vi "QTrkGenerateSampleFromLUT.vi"(0 "Width":i32=80, 1 "Height":i32=80, 2 "position":cluster{"x":sgl, "y":sgl}={"x"=40.0, "y"=40.0}, 3 "LUT":sgl[][](array[numeric]), 4 "magnification":sgl=1.0, 5 "LUT radii":cluster{"min":sgl, "max":sgl}={"min"=0.0, "max"=40.0}, 7 "z":sgl=10.0, 9 "photoncountpp":sgl) -> (14 "image":sgl[][](array[numeric]))   [LabVIEW 2011]
uses:
  QTrkDLL.vi
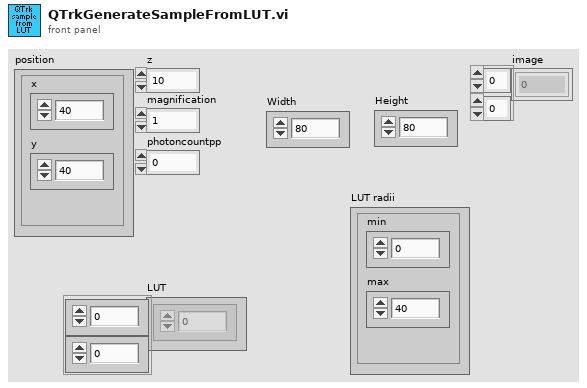
[diagram p1: front panel]
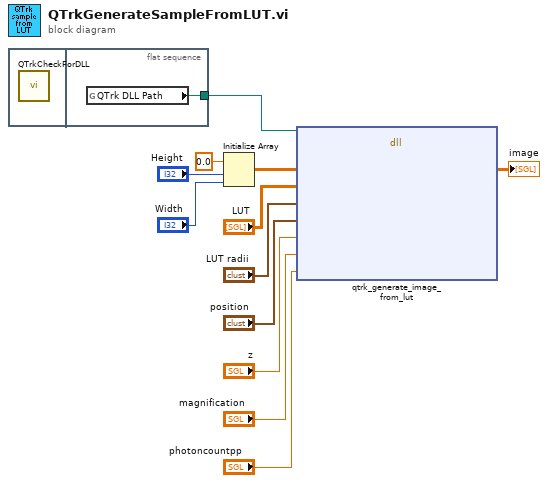
[diagram p0: block diagram]
diagram:
  n1 = flat-sequence {
    tunnel: [w13] -> w1
    frame #0 {
      n2 = call "QTrkCheckForDLL.vi"() -> ()  [unwired: 12 in]
    }
    frame #1 {
      n3 = global read "QTrkDLL.vi" "QTrk DLL Path"() -> (w13:path)
    }
  }
  n4 = Initialize Array(sgl 0.0 ("element"), "Height", "Width") -> (w8:sgl[][])
  n5 = dll-call lib="D:/jcnossen1/cudaqi-tracker/bin/jtrk-labview.dll" fn="qtrk_generate_image_from_lut"(path in=w1, "image"=w8, "lut"="LUT", "LUTradii"="LUT radii", "position"="position", "z"="z", "magnification"="magnification", "photoncountpp"="photoncountpp") -> ("image"=→"image":sgl[][])  [unwired: 9 in, 2 out]
